vi "Pre Launch Init.vi"(11 "PowerSupply in":refnum<class "PowerSupply.lvclass">) -> (0 "error out":errorcluster, 3 "PowerSupply out":refnum<class "PowerSupply.lvclass">)   [LabVIEW 2019, in "PowerSupply.lvlib" / "PowerSupply.lvclass"]
uses:
  Library/PowerSupply.lvclass
  builds/Instruments/Instruments.lvlibp/Library/Instruments.lvclass
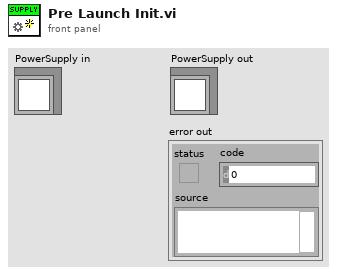
[diagram p1: front panel]
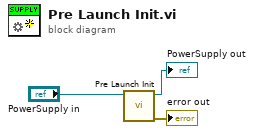
[diagram p0: block diagram]
diagram:
  n1 = call-parent "Pre Launch Init.vi"("Instruments in"="PowerSupply in") -> ("error out"=→"error out":errorcluster, "Instruments out"=→"PowerSupply out":refnum<class "PowerSupply.lvclass">)  [unwired: 9 in]
